vi "identify NML data acq version.vi"() -> (2 "NML data in the memory":string)   [LabVIEW 2020]
panel:
  in  "NML Data Acquisition VI":string(combo)="NML Data Acquisition-New.vi"
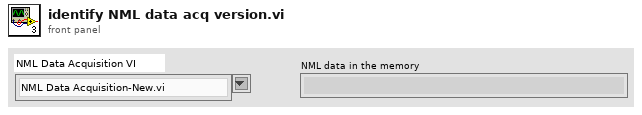
[diagram p1: front panel]
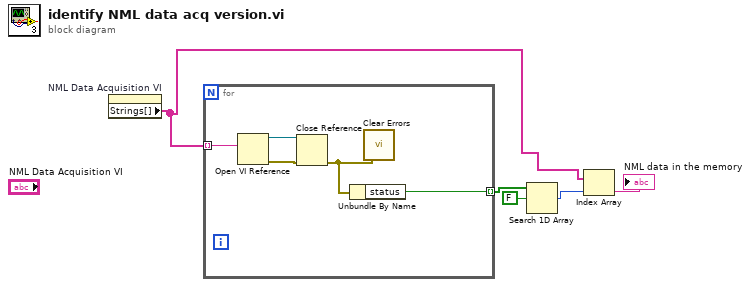
[diagram p0: block diagram]
diagram:
  n1 = property on="NML Data Acquisition VI" class="CmbBox"() -> ("Strings[]"=w2:string[])  [unwired: 2 in, 2 out]
  n2 = for {
    tunnel: w2 -> [w8] mode=indexing
    tunnel: [w6] -> w5 mode=indexing
    n3 = Open VI Reference(vi path=w8) -> (vi reference=w10:refnum<vi>, error out=w9:errorcluster)  [unwired: 1 in, 4 out]
    n4 = Close Reference(reference=w10, error in (no error)=w9) -> (error out=w7:errorcluster)
    n5 = Unbundle By Name(w7) -> ("status"=w6:bool)
    n6 = call <vilib>:"Clear Errors.vi"("error in (no error)"=w7) -> ()  [unwired: 5 in, 2 out]
  }
  n7 = Search 1D Array(1D array=w5, element=FALSE) -> (index of element=w3:i32)  [unwired: 1 in]
  n8 = Index Array(array=w2, index=w3) -> (element=→"NML data in the memory":string)
